vi "Read Array.vi"(6 "Value":string, 8 "Error In":errorcluster, 9 "Variant DB":variant, 10 "Name":string, 11 "Variant":variant) -> (0 "Error Out":errorcluster, 3 "String":string)   [LabVIEW 2020, in "Configit.lvlib"]
uses:
  Configit.lvlib
  <vilib>/Utility/VariantDataType/Type.ctl
  <vilib>/Waveform/DWDTOps.llb/DWDT Empty Digital.vi
  <vilib>/Waveform/DTblOps.llb/DTbl Empty Digital.vi
  <vilib>/Utility/VariantDataType/VariantType.lvlib
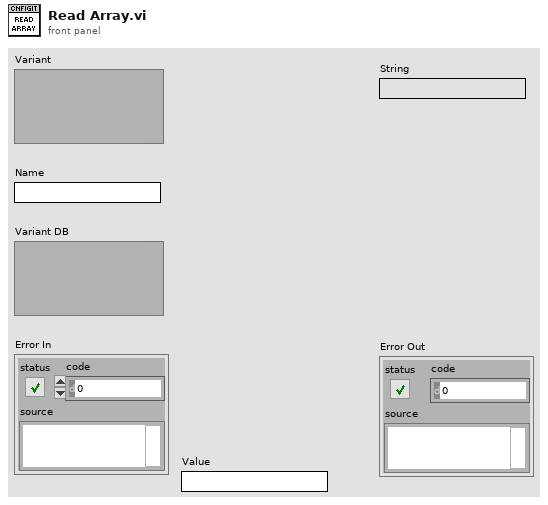
[diagram p1: front panel]
types:
  T1 = typedef "VariantType.lvlib/Type.ctl" = enum8{"Invalid Type", "Void", "I8", "I16", "I32", "I64", "U8", "U16", "U32", "U64", "Single Float", "Double Float", "Extended Float", "Single Complex", "Double Complex", "Extended Complex", "Enum U8", "Enum U16", "Enum U32", "Enum U64", "Single Float With Unit", "Double Float With Unit", "Extended Float With Unit", "Single Complex with Unit", "Double Complex with Unit", "Extended Complex with Unit", "Boolean", "String", "Path", "Picture", "Tag", "Array", "Cluster", "Variant", "LV Variant", "Waveform", "Timestamp", "Digital Waveform", "Digital Data", "ExpressData", "Refnum", "External Data", "VI", "Poly VI", "LabVIEW Class Instance", "Fixed Point"}
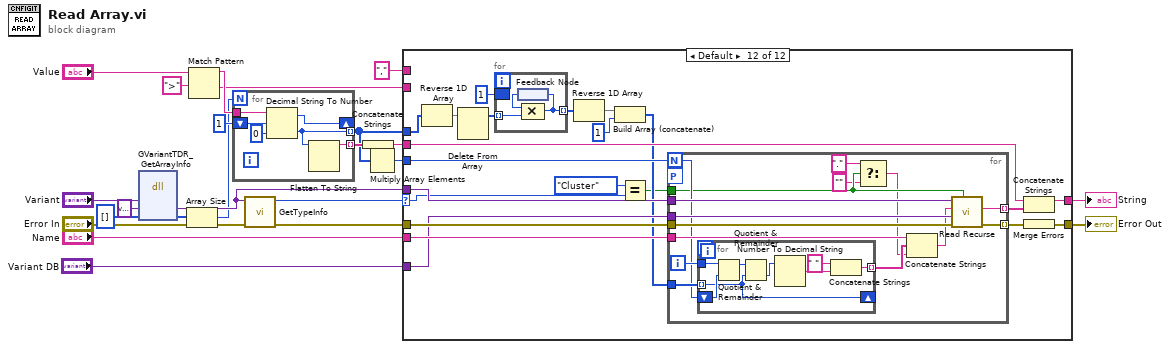
[diagram p0: block diagram]
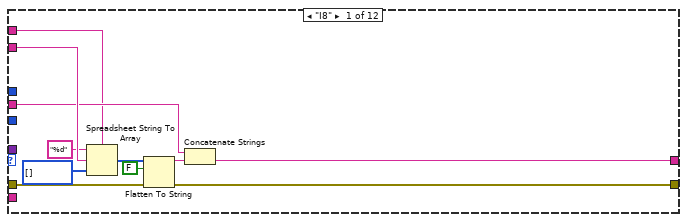
[diagram p2: hidden frame]
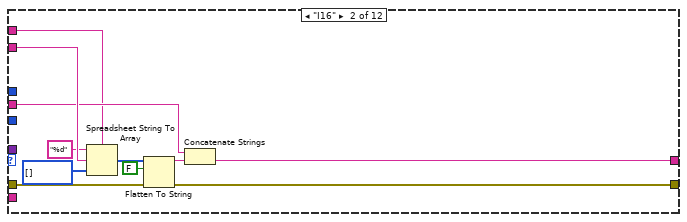
[diagram p3: hidden frame]
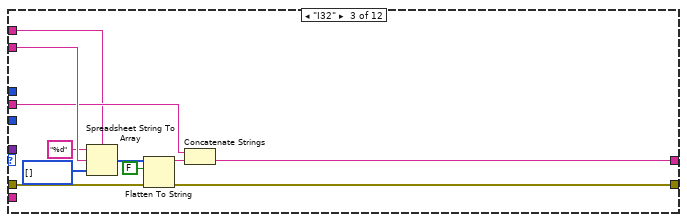
[diagram p4: hidden frame]
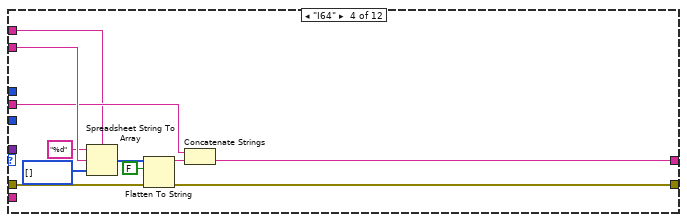
[diagram p5: hidden frame]
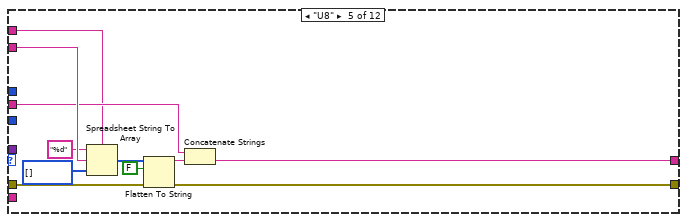
[diagram p6: hidden frame]
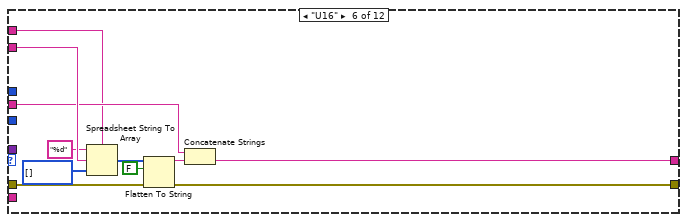
[diagram p7: hidden frame]
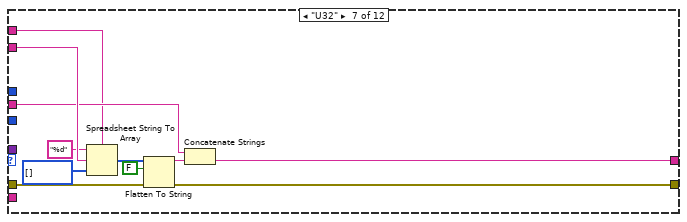
[diagram p8: hidden frame]
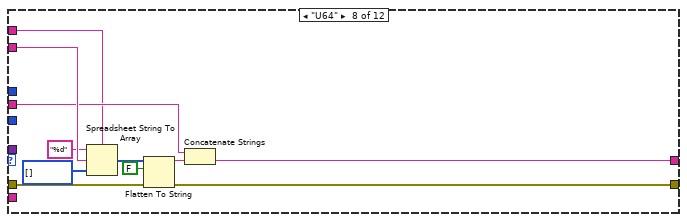
[diagram p9: hidden frame]
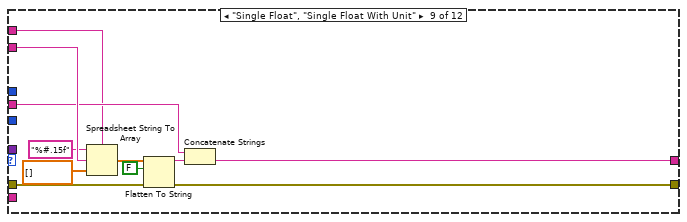
[diagram p10: hidden frame]
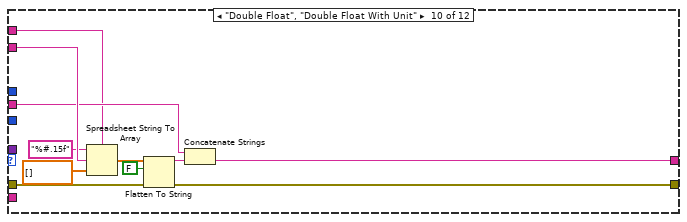
[diagram p11: hidden frame]
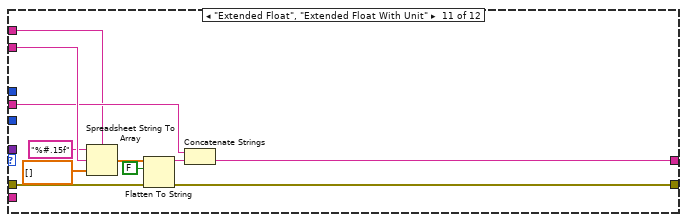
[diagram p12: hidden frame]
diagram:
  n1 = dll-call lib="LabVIEW" fn="GVariantTDR_GetArrayInfo"("lvVar"="Variant", "eltType"=variant ("ArrayElt"), "dimInfo"=i32[] []) -> ("eltType"=w3:variant, "dimInfo"=w2:i32[])  [unwired: 5 in, 2 out]
  n2 = Array Size(array=w2) -> (size(s)=w1:i32)
  n3 = Match Pattern(string="Value", regular expression=">") -> (before substring=w20:string, after substring=w16:string)  [unwired: 1 in, 2 out]
  n4 = for {
    N: w1 -> [_]
    shift-right: [w28] -> _
    shift-left: 1 ("offset past number") -> [w27]
    tunnel: w20 -> [w29]
    tunnel: [w25] -> w9 mode=indexing
    tunnel: [w24] -> w22 mode=indexing
    n5 = Decimal String To Number(string=w29, offset=w27, default (0L)=u32 0 ("default (0 I32)")) -> (offset past number=w28:i32, number=w25:u32)
    n6 = Flatten To String(anything=w25) -> (data string=w24:string)  [unwired: 3 in, 2 out]
  }
  n7 = call "GetTypeInfo.vi"("Error In"="Error In", "Variant"=w3) -> ("Error Out"=w17:errorcluster, "Type Enum"=w18:T1)  [unwired: 6 in, 2 out]
  n8 = Concatenate Strings(w22) -> (w15:string)
  n9 = Multiply Array Elements(1:w9) -> (0:w10:u32)
  n10 = case shown="Default" w18 {
    selector: w18 -> [_ _ _ _ _ _ _ _ _ _ _ w154]
    tunnel: w17 -> [w36 w47 w58 w69 w80 w91 w102 w113 w124 w135 w146 w171]
    tunnel: w16 -> [w35 w46 w57 w68 w79 w90 w101 w112 w123 w134 w145 _]
    tunnel: w15 -> [w33 w44 w55 w66 w77 w88 w99 w110 w121 w132 w143 w164]
    tunnel: [w32 w43 w54 w65 w76 w87 w98 w109 w120 w131 w142 w151] -> w14
    tunnel: [w31 w42 w53 w64 w75 w86 w97 w108 w119 w130 w141 w165] -> w13
    tunnel: w3 -> [_ _ _ _ _ _ _ _ _ _ _ w169]
    tunnel: "Name" -> [_ _ _ _ _ _ _ _ _ _ _ w167]
    tunnel: "Variant DB" -> [_ _ _ _ _ _ _ _ _ _ _ w166]
    tunnel: w10 -> [_ _ _ _ _ _ _ _ _ _ _ w163]
    tunnel: w9 -> [_ _ _ _ _ _ _ _ _ _ _ w157]
    tunnel: "," ("delimiter (Tab)") -> [w30 w41 w52 w63 w74 w85 w96 w107 w118 w129 w140 _]
    frame "I8" {
      n11 = Spreadsheet String To Array(delimiter (Tab)=w30, format string="%d", spreadsheet string=w35, array type (2D Dbl)=i8[] []) -> (array=w40:i8[])
      n12 = Flatten To String(anything=w40, prepend array or string size? (T)=FALSE, error in (no error)=w36) -> (data string=w37:string, error out=w32:errorcluster)  [unwired: 1 in, 1 out]
      n13 = Concatenate Strings(w33, w37) -> (w31:string)
    }
    frame "I16" {
      n14 = Spreadsheet String To Array(delimiter (Tab)=w41, format string="%d", spreadsheet string=w46, array type (2D Dbl)=i16[] []) -> (array=w51:i16[])
      n15 = Flatten To String(anything=w51, prepend array or string size? (T)=FALSE, error in (no error)=w47) -> (data string=w48:string, error out=w43:errorcluster)  [unwired: 1 in, 1 out]
      n16 = Concatenate Strings(w44, w48) -> (w42:string)
    }
    frame "I32" {
      n17 = Spreadsheet String To Array(delimiter (Tab)=w52, format string="%d", spreadsheet string=w57, array type (2D Dbl)=i32[] []) -> (array=w62:i32[])
      n18 = Flatten To String(anything=w62, prepend array or string size? (T)=FALSE, error in (no error)=w58) -> (data string=w59:string, error out=w54:errorcluster)  [unwired: 1 in, 1 out]
      n19 = Concatenate Strings(w55, w59) -> (w53:string)
    }
    frame "I64" {
      n20 = Spreadsheet String To Array(delimiter (Tab)=w63, format string="%d", spreadsheet string=w68, array type (2D Dbl)=i64[] []) -> (array=w73:i64[])
      n21 = Flatten To String(anything=w73, prepend array or string size? (T)=FALSE, error in (no error)=w69) -> (data string=w70:string, error out=w65:errorcluster)  [unwired: 1 in, 1 out]
      n22 = Concatenate Strings(w66, w70) -> (w64:string)
    }
    frame "U8" {
      n23 = Spreadsheet String To Array(delimiter (Tab)=w74, format string="%d", spreadsheet string=w79, array type (2D Dbl)=u8[] []) -> (array=w84:u8[])
      n24 = Flatten To String(anything=w84, prepend array or string size? (T)=FALSE, error in (no error)=w80) -> (data string=w81:string, error out=w76:errorcluster)  [unwired: 1 in, 1 out]
      n25 = Concatenate Strings(w77, w81) -> (w75:string)
    }
    frame "U16" {
      n26 = Spreadsheet String To Array(delimiter (Tab)=w85, format string="%d", spreadsheet string=w90, array type (2D Dbl)=u16[] []) -> (array=w95:u16[])
      n27 = Flatten To String(anything=w95, prepend array or string size? (T)=FALSE, error in (no error)=w91) -> (data string=w92:string, error out=w87:errorcluster)  [unwired: 1 in, 1 out]
      n28 = Concatenate Strings(w88, w92) -> (w86:string)
    }
    frame "U32" {
      n29 = Spreadsheet String To Array(delimiter (Tab)=w96, format string="%d", spreadsheet string=w101, array type (2D Dbl)=u32[] []) -> (array=w106:u32[])
      n30 = Flatten To String(anything=w106, prepend array or string size? (T)=FALSE, error in (no error)=w102) -> (data string=w103:string, error out=w98:errorcluster)  [unwired: 1 in, 1 out]
      n31 = Concatenate Strings(w99, w103) -> (w97:string)
    }
    frame "U64" {
      n32 = Spreadsheet String To Array(delimiter (Tab)=w107, format string="%d", spreadsheet string=w112, array type (2D Dbl)=u64[] []) -> (array=w117:u64[])
      n33 = Flatten To String(anything=w117, prepend array or string size? (T)=FALSE, error in (no error)=w113) -> (data string=w114:string, error out=w109:errorcluster)  [unwired: 1 in, 1 out]
      n34 = Concatenate Strings(w110, w114) -> (w108:string)
    }
    frame "Single Float", "Single Float With Unit" {
      n35 = Spreadsheet String To Array(delimiter (Tab)=w118, format string="%#.15f", spreadsheet string=w123, array type (2D Dbl)=sgl[] []) -> (array=w128:sgl[])
      n36 = Flatten To String(anything=w128, prepend array or string size? (T)=FALSE, error in (no error)=w124) -> (data string=w125:string, error out=w120:errorcluster)  [unwired: 1 in, 1 out]
      n37 = Concatenate Strings(w121, w125) -> (w119:string)
    }
    frame "Double Float", "Double Float With Unit" {
      n38 = Spreadsheet String To Array(delimiter (Tab)=w129, format string="%#.15f", spreadsheet string=w134, array type (2D Dbl)=dbl[] []) -> (array=w139:dbl[])
      n39 = Flatten To String(anything=w139, prepend array or string size? (T)=FALSE, error in (no error)=w135) -> (data string=w136:string, error out=w131:errorcluster)  [unwired: 1 in, 1 out]
      n40 = Concatenate Strings(w132, w136) -> (w130:string)
    }
    frame "Extended Float", "Extended Float With Unit" {
      n41 = Spreadsheet String To Array(delimiter (Tab)=w140, format string="%#.15f", spreadsheet string=w145, array type (2D Dbl)=ext[] []) -> (array=w150:ext[])
      n42 = Flatten To String(anything=w150, prepend array or string size? (T)=FALSE, error in (no error)=w146) -> (data string=w147:string, error out=w142:errorcluster)  [unwired: 1 in, 1 out]
      n43 = Concatenate Strings(w143, w147) -> (w141:string)
    }
    frame Default {
      n44 = Reverse 1D Array(array=w157) -> (reversed array=w158:u32[])
      n45 = Delete From Array(array=w158) -> (array with subset deleted=w159:u32[])  [unwired: 2 in, 1 out]
      n46 = for {
        tunnel: w159 -> [w174] mode=indexing
        tunnel: [w172] -> w161 mode=indexing
        border: u32 1 -> [_]
        n47 = feedback #1() -> (w173:u32)
        n48 = Compound Arithmetic op=MULTIPLY(w173, w174) -> (w172:u32)
        n49 = feedback-in #1(w172) -> ()
      }
      n50 = Reverse 1D Array(array=w161) -> (reversed array=w162:u32[])
      n51 = Build Array (concatenate)(w162, u32 1) -> (w155:u32[])
      n52 = Equal?(x=Type."Cluster", y=w154) -> (x = y?=w152:bool)
      n53 = for {
        N: w163 -> [w180]
        tunnel: w169 -> [w187]
        tunnel: [w186] -> w168 mode=indexing
        tunnel: w167 -> [w184]
        tunnel: w166 -> [w185]
        tunnel: w155 -> [w181]
        tunnel: w152 -> [w178]
        workers-P: _ -> [_]
        tunnel: w171 -> [w189]
        tunnel: [w188] -> w170 mode=indexing
        i -> [w182]
        n54 = for {
          tunnel: [w196] -> w179 mode=indexing
          tunnel: w182 -> [w194]
          tunnel: w181 -> [w190] mode=indexing
          shift-right: [w190] -> _
          shift-left: w180 -> [w191]
          n55 = Quotient & Remainder(x=w194, y=w191) -> (x-y*floor(x/y)=w195:u32)  [unwired: 1 out]
          n56 = Quotient & Remainder(x=w195, y=w190) -> (floor(x/y)=w193:u32)  [unwired: 1 out]
          n57 = Number To Decimal String(number=w193) -> (decimal integer string=w197:string)  [unwired: 1 in]
          n58 = Concatenate Strings(" " ("string"), w197) -> (w196:string)
        }
        n59 = Select(t="." ("string"), s=w178, f="") -> (s? t:f=w176:string)
        n60 = Concatenate Strings(w184, w179, w176) -> (w183:string)
        n61 = call "Read Recurse.vi"("Append Name (T)"=w178, "Error In"=w189, "Variant DB"=w185, "Name"=w183, "Variant"=w187) -> ("Error Out"=w188:errorcluster, "String"=w186:string)  [unwired: 5 in]
      }
      n62 = Concatenate Strings(w164, w168) -> (w165:string)
      n63 = Merge Errors(w170) -> (w151:errorcluster)
    }
  }
  "Error Out" <- w14
  "String" <- w13
